vi "uNotify TruncateClassName.vi"(8 "error in (no error)":errorcluster, 10 "LV Class Name in":string) -> (0 "error out":errorcluster, 2 "LV Class Name out":string)   [LabVIEW 2021, in "uFramework.lvlib" / "uNotifyMode.lvclass"]
doc: "Remove from the LV class name string any of the following extensions:\n.lvclass\n.lvlibp\n.lvlib"
uses:
  uNotifyMode.lvclass
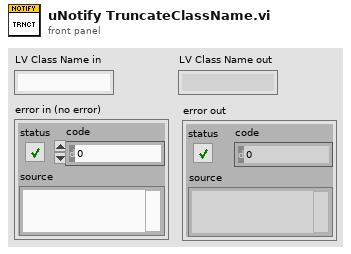
[diagram p1: front panel]
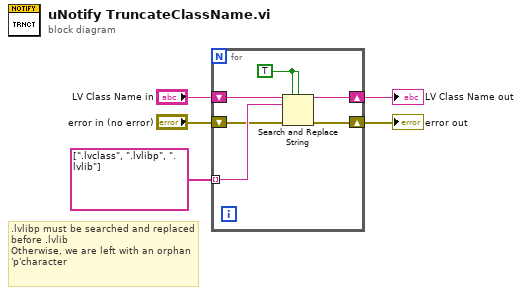
[diagram p0: block diagram]
diagram:
  # ".lvlibp must be searched and replaced before .lvlib\nOtherwise, we are left with an orphan 'p'character"
  n1 = for {
    tunnel: string[] [".lvclass", ".lvlibp", ".lvlib"] ("search string") -> [w9] mode=indexing
    shift-right: [w8] -> w3
    shift-left: "LV Class Name in" -> [w10]
    shift-right: [w6] -> w1
    shift-left: "error in (no error)" -> [w7]
    w11 = TRUE ("replace all? (F)")
    n2 = Search and Replace String(replace all?=w11, case sensitive?=w11, input string=w10, search string=w9, error in=w7) -> (result string=w8:string, error out=w6:errorcluster)  [unwired: 3 in, 2 out]
  }
  "LV Class Name out" <- w3
  "error out" <- w1
